vi "Merge Error.vi"(10 "Error":errorcluster, 11 "Base Event in":refnum<class "Base Event.lvclass">) -> (3 "Base Event out":refnum<class "Base Event.lvclass">)   [LabVIEW 2021, in "jettl.lvlib" / "Base Event.lvlib" / "Base Event.lvclass"]
uses:
  Base Event.lvclass
  Base Event.lvclass/Base Event.ctl
  State/Error State/Error State.lvclass
  C:/git/jettl/jettl/jettl/Base Event/State/State/State.lvclass
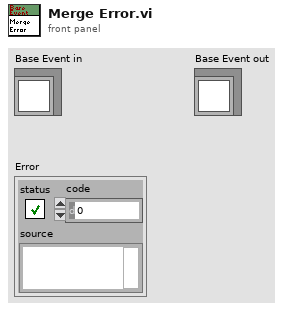
[diagram p1: front panel]
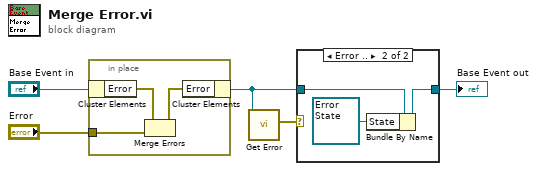
[diagram p0: block diagram]
diagram:
  n1 = in-place {
    in-place-border: "Error" -> [w6]
    n2 = in-place-cluster #1("Base Event in") -> ("Error"=w8:errorcluster)
    n3 = Merge Errors(w8, w6) -> (w7:errorcluster)
    n4 = in-place-cluster #1("Error"=w7) -> (w2:refnum<class "Base Event.lvclass">)
  }
  n5 = call-dynamic "Get Error.vi"("Base Event in"=w2) -> ("Error"=w3:errorcluster)  [unwired: 10 in]
  n6 = case shown="Error .." w3 {
    tunnel: [w9 w11] -> w1
    tunnel: w2 -> [w9 w12]
    frame No Error {
    }
    frame Error {
      n7 = Bundle By Name(cluster=w12, "State"=refnum<class "Error State.lvclass"> refnum ("jettl.lvlib:Error Event State.lvclass")) -> (w11:refnum<class "Base Event.lvclass">)
    }
  }
  "Base Event out" <- w1
